vi "Register (async).vi"(0 "WAMP Client in":refnum<class "WAMP Client.lvclass">, 1 "Options":string, 5 "Procedure URI":string, 11 "error in (no error)":errorcluster) -> (4 "WAMP Client out":refnum<class "WAMP Client.lvclass">, 8 "Result notifier":refnum<notifier>, 15 "error out":errorcluster)   [LabVIEW 2020, in "wamplv.lvlib" / "WAMP Client.lvclass"]
uses:
  WAMP Client.lvclass
  TypeDef/Success or error.ctl
  API/TypeDefs/Combined error.ctl
  API/TypeDefs/WAMP error.ctl
  TypeDef/REGISTER Request Data.ctl
  TypeDef/Internal Message Type.ctl
  WAMP Client.lvclass/WAMP Client.ctl
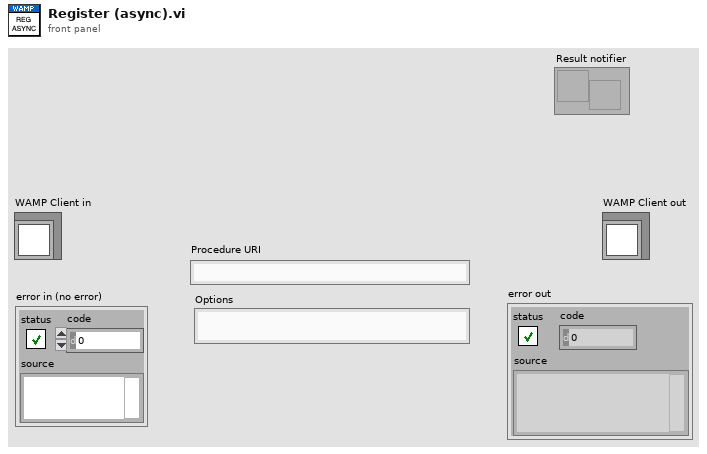
[diagram p1: front panel]
types:
  T1 = typedef "wamplv.lvlib/WAMP Client.lvclass/Success or error.ctl" = cluster{"Success?":bool, "URI":string, "Combined Error":T2}
  T2 = typedef "wamplv.lvlib/WAMP Client.lvclass/Combined error.ctl" = cluster{"Error?":bool, "WAMP Error":T3, "Error":errorcluster}
  T3 = typedef "wamplv.lvlib/WAMP Client.lvclass/WAMP error.ctl" = cluster{"Details":string, "ArgumentKw Payload":string, "Error?":bool, "Error URI":string, "Arguments Payload":string}
  T4 = typedef "wamplv.lvlib/WAMP Client.lvclass/Internal Message Type.ctl" = enum16{"Subscribe", "Handle Subscribed", "Handle Event", "Unsubscribe", "Handle Unsubscribed", "Publish", "Handled Published", "Goodbye", "Handle Goodbye", "Call", "Handle Result", "Register", "Handle Registered", "Unregister", "Handle Unregistered", "Handle Invocation", "Yield", "Error"}
  T5 = typedef "wamplv.lvlib/WAMP Client.lvclass/REGISTER Request Data.ctl" = cluster{"Procedure URI":string, "Options":string, "REGISTER result notifier":refnum<notifier>}
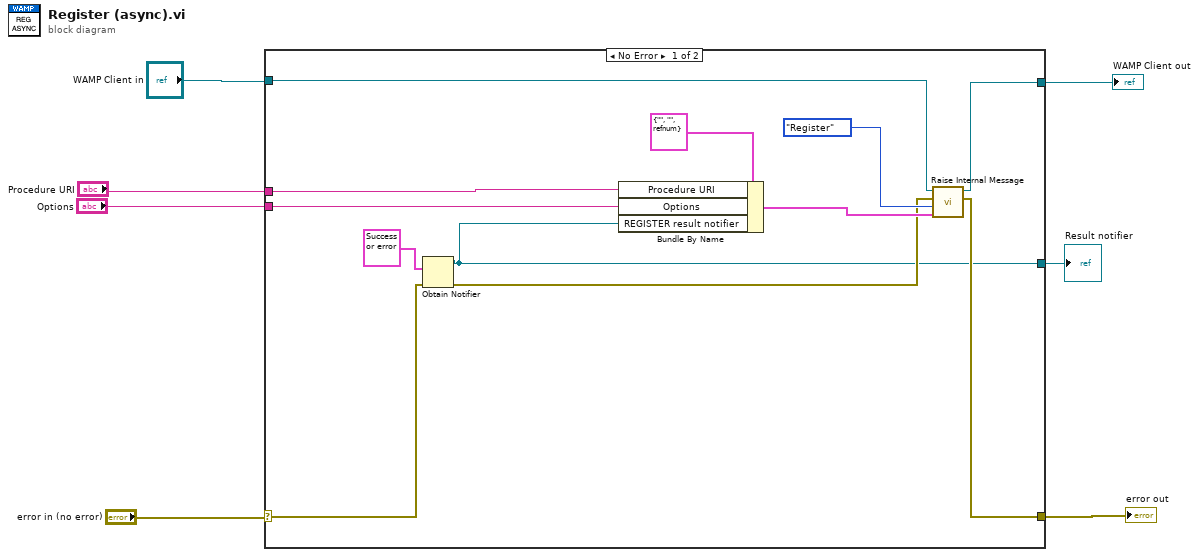
[diagram p0: block diagram]
diagram:
  n1 = case shown="No Error" "error in (no error)" {
    selector: "error in (no error)" -> [w8 w21]
    tunnel: [w12 w21] -> w6
    tunnel: [w15 w20] -> w4
    tunnel: "WAMP Client in" -> [w16 w20]
    tunnel: "Procedure URI" -> [w18 _]
    tunnel: "Options" -> [w17 _]
    tunnel: [w9 _] -> w1
    frame No Error {
      n2 = Obtain Notifier(notification data type=T1 {"Success?"=FALSE, "URI"="", "Combined Error"={"Error?"=FALSE, "WAMP Error"={"Details"="{}", "ArgumentKw Payload"="", "Error?"=FALSE, "Error URI"="", "Arguments Payload"=""}, "Error"={"status"=FALSE, "code"=0, "source"=""}}} ("REGISTERED or ERROR payload"), error in (no error)=w8) -> (notifier out=w9:refnum<notifier>, error out=w10:errorcluster)  [unwired: 2 in, 1 out]
      n3 = Bundle By Name(cluster=T5 {"Procedure URI"="", "Options"="", "REGISTER result notifier"=refnum} ("REGISTER request data"), "Procedure URI"=w18, "Options"=w17, "REGISTER result notifier"=w9) -> (w13:T5)
      n4 = call-dynamic "Raise Internal Message.vi"("Variant"=w13, "Internal Message Type"=Internal_Message_Type."Register", "error in (no error)"=w10, "WAMP Client in"=w16) -> ("error out"=w12:errorcluster, "WAMP Client out"=w15:refnum<class "WAMP Client.lvclass">)  [unwired: 6 in]
    }
    frame Error {
    }
  }
  "error out" <- w6
  "WAMP Client out" <- w4
  "Result notifier" <- w1
